vi "Event Input Snip.vi"() -> ()   [LabVIEW 2015]
uses:
  Event Input/Event Input.lvclass/Event Input.ctl
  Result/result.lvclass/result.ctl
  Result/result.lvclass
  Event Input/Event Input.lvclass
  Input/input.lvclass
panel:
  in  "Stop Button":bool
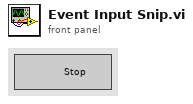
[diagram p1: front panel]
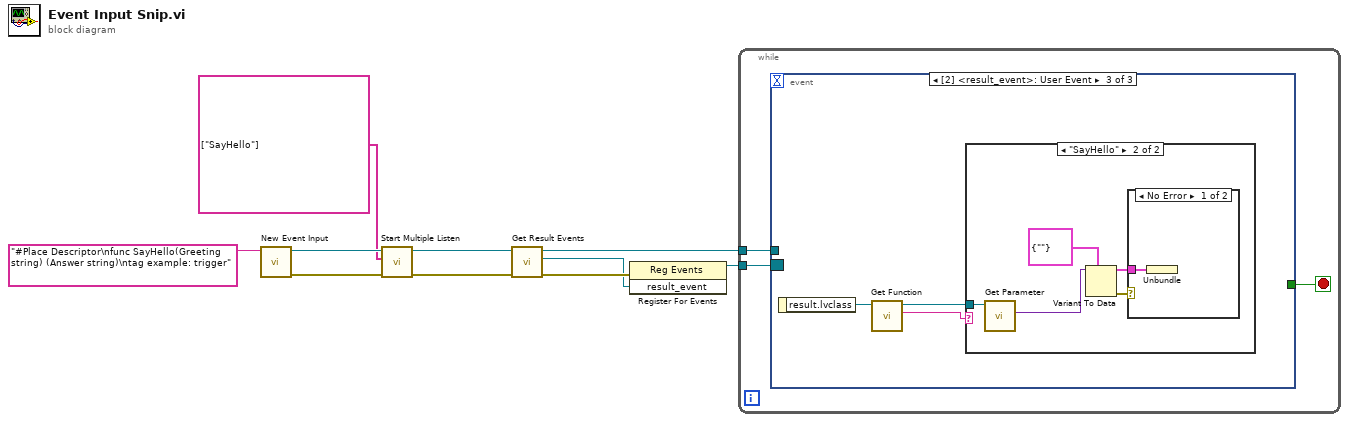
[diagram p0: block diagram]
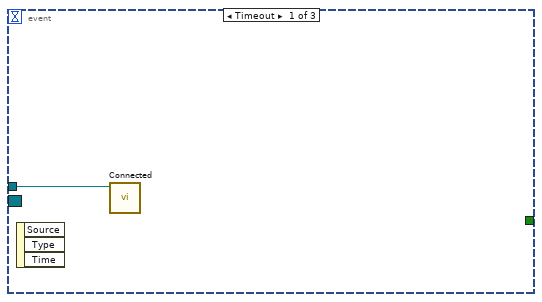
[diagram p2: hidden frame]
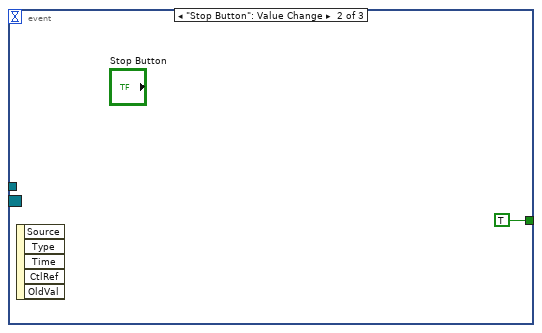
[diagram p3: hidden frame]
diagram:
  n1 = call "New Event Input.vi"("Descriptor"="#Place Descriptor\nfunc SayHello(Greeting string) (Answer string)\ntag example: trigger") -> ("error out"=w8:errorcluster, "event_input out"=w9:refnum<class "Event Input.lvclass">)  [unwired: 9 in]
  n2 = call "Start Multiple Listen.vi"("error in (no error)"=w8, "Functions"=string[] ["SayHello"], "input in"=w9) -> ("error out"=w5:errorcluster, "input out"=w6:refnum<class "Event Input.lvclass">)  [unwired: 7 in]
  n3 = call "Get Result Events.vi"("error in (no error)"=w5, "event_input in"=w6) -> ("error out"=w4:errorcluster, "result_event"=w3:refnum<user-event>, "event_input out"=w1:refnum<class "Event Input.lvclass">)  [unwired: 7 in]
  n4 = register-events(error in=w4, w3) -> (reference out=w2:refnum<event-registration>)  [unwired: 1 in, 1 out]
  n5 = while {
    tunnel: w2 -> [w12]
    tunnel: w1 -> [w11]
    stop <- w13 stop-if-true
    n6 = event shown="[2] <result_event>: User Event" {
      selector: w12 -> [_ _ _]
      dyn-events: _ -> [_ _ _]
      timeout: _ -> [_ _ _]
      tunnel: [_ TRUE _] -> w13
      tunnel: w11 -> [w14 _ _]
      event Timeout {
        n7 = event-data() -> ()  [unwired: 1 in, 3 out]
        n8 = call "Connected.vi"("input in"=w14) -> ()  [unwired: 8 in, 3 out]
      }
      event "Stop Button": Value Change {
        n9 = event-data() -> ()  [unwired: 1 in, 5 out]
      }
      event User Event {
        n10 = event-data() -> ("result.lvclass"=w18:refnum<class "result.lvclass">)  [unwired: 1 in]
        n11 = call "Get Function.vi"("result in"=w18) -> ("function"=w17:string, "result out"=w16:refnum<class "result.lvclass">)  [unwired: 8 in, 1 out]
        n12 = case shown="\"SayHello\"" w17 {
          tunnel: w16 -> [_ w23]
          frame Default {
          }
          frame "SayHello" {
            n13 = call-dynamic "Get Parameter.vi"("result in"=w23) -> ("Data"=w22:variant)  [unwired: 8 in, 2 out]
            n14 = Variant To Data(type=cluster{"Answer":string} {"Answer"=""}, Variant=w22) -> (data=w20:cluster{"Answer":string}, error out=w19:errorcluster)  [unwired: 1 in]
            n15 = case shown="No Error" w19 {
              tunnel: w20 -> [w24 _]
              frame No Error {
                n16 = Unbundle(w24) -> ()  [unwired: 1 out]
              }
              frame Error {
              }
            }
          }
        }
      }
    }
  }
